vi "ReadFile.vi"(0 "File Path":path, 5 "Error In":errorcluster) -> (14 "file path":path, 15 "Initialize Settings":T1, 16 "Channel(s) Settings":T4 {"Channel(s)"."Verticle Settings"."Vertical Coupling" items=["AC", "DC", "Ground"]; "Channel(s)"."Verticle Settings"."Probe Attenuation" format="%.1f"; "Channel(s)"."Verticle Settings"."Vertical Offset" format="%.2p"; "Channel(s)"."Verticle Settings"."Vertical Range" format="%.2f"; "Channel(s)"."Maximum Input Frequency" format="%.2f"}, 17 "Specific&CommonTriggerProperties":T3={"Common Trigger Settings"={"Trigger Delay"=0.0, "Reference Position"=50.0, "Trigger Modifier"=2, "Auto Triggered"=FALSE}, "Specific Trigger Settings"={"Source"="", "Holdoff"=0.0, "Level"=0.0, "Trigger Slope"=enum."Negative", "Type"=enum."Immediate", "Window Mode"=0, "Low Level"=-0.1, "High Level"=0.1, "Coupling"=1, "Hysteresis"=0.05}} {"Specific Trigger Settings"."Hysteresis" format="%.2f"; "Specific Trigger Settings"."Coupling" items=["AC"=0, "DC"=1, "HF Reject"=3, "LF Reject"=4, "AC Plus HF Reject"=1001]; "Specific Trigger Settings"."High Level" format="%.2f"; "Specific Trigger Settings"."Low Level" format="%.2f"; "Specific Trigger Settings"."Window Mode" items=["Entering", "Leaving"]; "Common Trigger Settings"."Trigger Modifier" items=["None"=1, "Auto Trigger"=2]; "Common Trigger Settings"."Reference Position" format="%.1f"; "Common Trigger Settings"."Trigger Delay" format="%#.4p"}, 18 "Horizontal Settings":T2={"Continuous"=FALSE, "EnableAveraging"=FALSE, "Number Averages"=0, "Measurement Timeout"=0.0, "Min Record Length"=1000, "Min Sample Rate"=10000000.0, "Enforce Realtime"=TRUE, "Sampling Mode "=enum."Real Time", "Interpolation"=enum."No Interpolation", "Type"=enum."Normal", "StartTime"=0.0, "Time Per Record"=0.0, "Number of Points Minimum"=0, "Measurement Name"="Sensor.RoomAlert0", "Measurement RefreshTime (ms)"=1000} {"Min Sample Rate" step=1000000.0 format="%#.2p"}, 19 "error out":errorcluster)   [LabVIEW 2018, in "ScopePlugins.lvlib" / "ScopePluginsBase.lvclass"]
uses:
  ScopePluginsBase.lvclass
  Typedefs/ChannelSetting(s).ctl
  Typedefs/TriggerSettings.ctl
  Typedefs/HorizontalSettings.ctl
  Typedefs/InitializationSettings.ctl
  <vilib>/Utility/config.llb/NI_LVConfig.lvlib
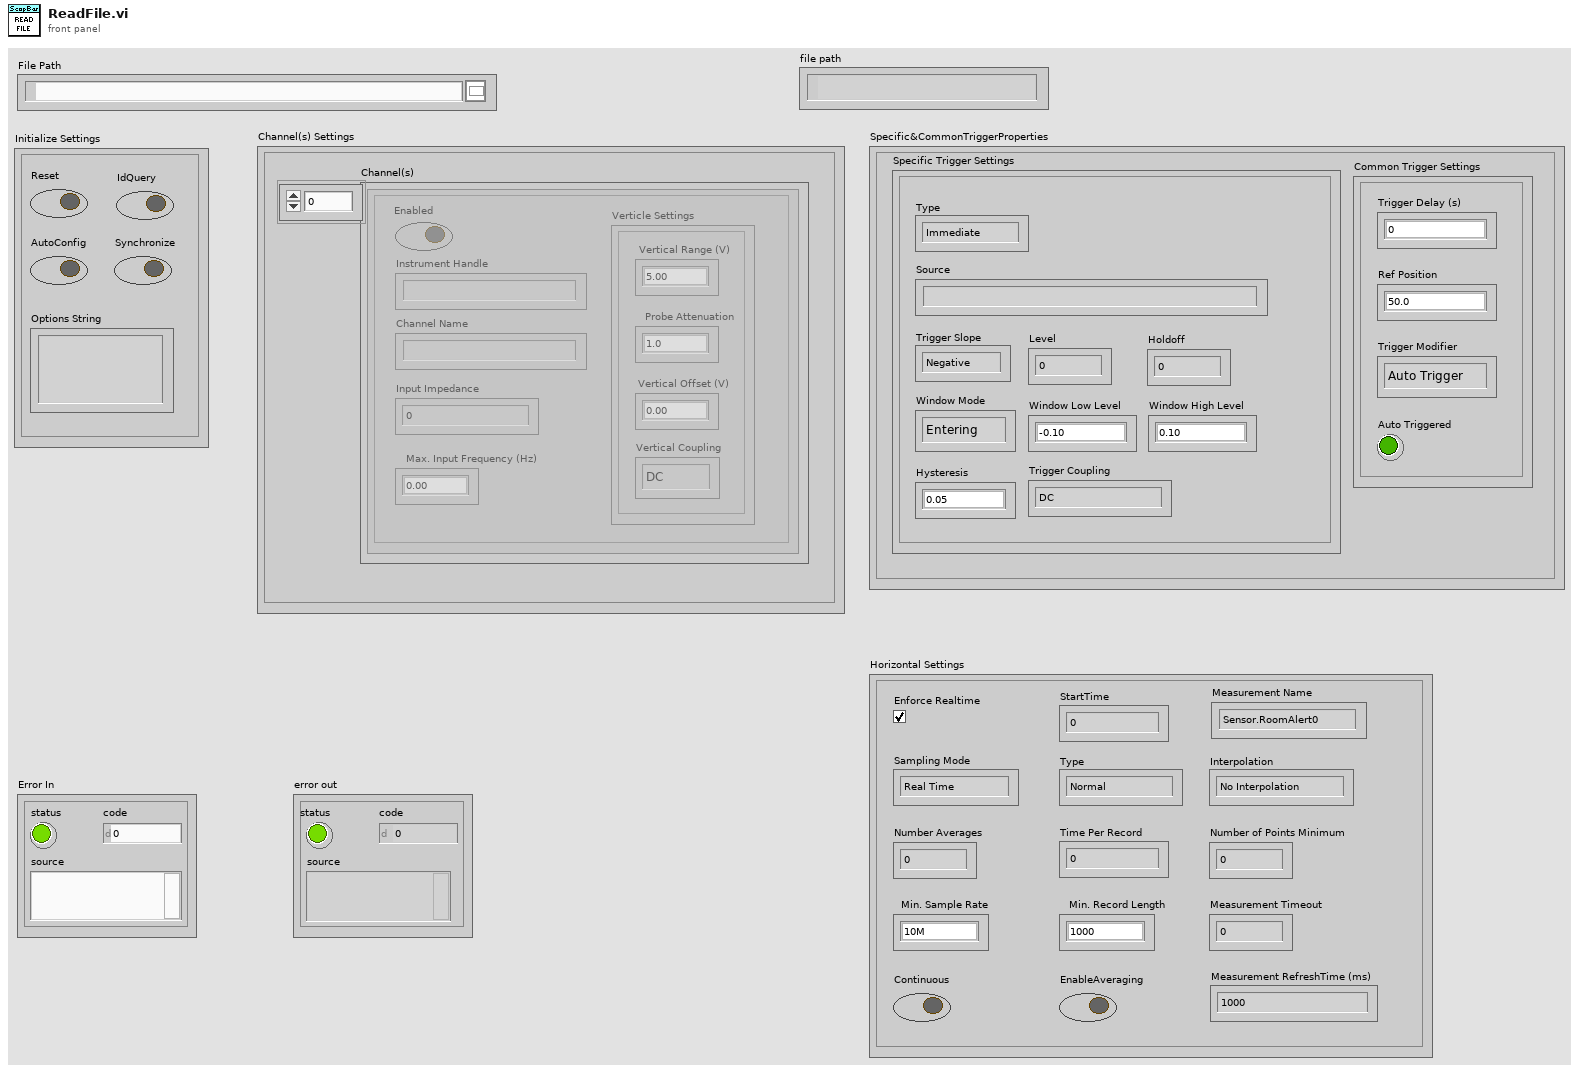
[diagram p1: front panel]
types:
  T1 = typedef "ScopePlugins.lvlib/ScopePluginsBase.lvclass/InitializationSettings.ctl" = cluster{"Reset":bool, "IdQuery":bool, "AutoConfig":bool, "Options String":string, "Synchronize":bool}
  T2 = typedef "ScopePlugins.lvlib/ScopePluginsBase.lvclass/HorizontalSettings.ctl" = cluster{"Continuous":bool, "EnableAveraging":bool, "Number Averages":i32, "Measurement Timeout":dbl, "Min Record Length":i32, "Min Sample Rate":dbl, "Enforce Realtime":bool, "Sampling Mode ":enum16{"Real Time", "Equivalent Time", "Segment", "Real Time Peak Detect", "Real Time High Resolution", "Peak Detect Segment", "High Resolution Segment"}, "Interpolation":enum16{"No Interpolation", "sin(x)/x", "linear", "1 Point sin(x)/x", "2 Point sin(x)/x", "4 Point sin(x)/x", "8 Point sin(x)/x", "16 Point sin(x)/x"}, "Type":enum16{"Normal", "PeakDetect", "HighRes", "Envelope", "Average"}, "StartTime":dbl, "Time Per Record":dbl, "Number of Points Minimum":i32, "Measurement Name":string, "Measurement RefreshTime (ms)":u32}
  T3 = typedef "ScopePlugins.lvlib/ScopePluginsBase.lvclass/TriggerSettings.ctl" = cluster{"Common Trigger Settings":cluster{"Trigger Delay":dbl, "Reference Position":dbl, "Trigger Modifier":i32, "Auto Triggered":bool}, "Specific Trigger Settings":cluster{"Source":string, "Holdoff":dbl, "Level":dbl, "Trigger Slope":enum16{"Negative", "Positive"}, "Type":enum16{"Immediate", "Edge", "Digitial", "Window", "Hysteresis", "Width", "Runt", "Glitch", "TV", "AC Line"}, "Window Mode":i32, "Low Level":dbl, "High Level":dbl, "Coupling":u16, "Hysteresis":dbl}}
  T4 = typedef "ScopePlugins.lvlib/ScopePluginsBase.lvclass/ChannelSetting(s).ctl" = cluster{"Number of Channels":i32, "Channel(s)":cluster{"Enabled":bool, "Instrument Handle":string, "Channel Name":string, "Maximum Input Frequency":dbl, "Verticle Settings":cluster{"Vertical Range":dbl, "Vertical Offset":dbl, "Probe Attenuation":dbl, "Vertical Coupling":i32}, "Connected":bool, "Input Impedance":dbl, "IO Type Instrument Handle":refnum<k15>}[]}
  T5 = typedef "NI_LVConfig.lvlib/Config Data RefNum.ctl" = refnum<k1>
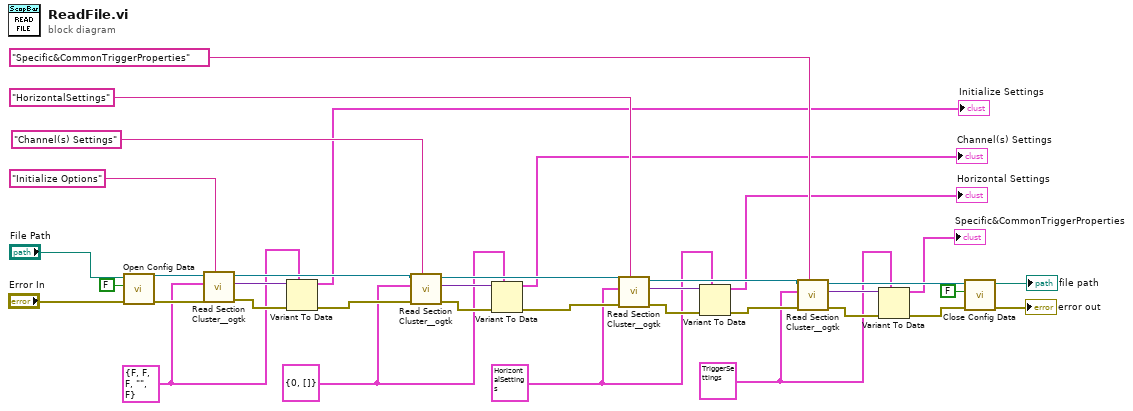
[diagram p0: block diagram]
diagram:
  w1 = T1 {"Reset"=FALSE, "IdQuery"=FALSE, "AutoConfig"=FALSE, "Options String"="", "Synchronize"=FALSE} ("Initialize Settings")
  w6 = T3 {"Common Trigger Settings"={"Trigger Delay"=0.0, "Reference Position"=50.0, "Trigger Modifier"=2, "Auto Triggered"=FALSE}, "Specific Trigger Settings"={"Source"="", "Holdoff"=0.0, "Level"=0.0, "Trigger Slope"=enum."Negative", "Type"=enum."Immediate", "Window Mode"=0, "Low Level"=-0.1, "High Level"=0.1, "Coupling"=1, "Hysteresis"=0.05}} ("Specific&CommonTriggerProperties")
  w7 = T2 {"Continuous"=FALSE, "EnableAveraging"=FALSE, "Number Averages"=0, "Measurement Timeout"=0.0, "Min Record Length"=1000, "Min Sample Rate"=10000000.0, "Enforce Realtime"=TRUE, "Sampling Mode "=enum."Real Time", "Interpolation"=enum."No Interpolation", "Type"=enum."Normal", "StartTime"=0.0, "Time Per Record"=0.0, "Number of Points Minimum"=0, "Measurement Name"="Sensor.RoomAlert0", "Measurement RefreshTime (ms)"=1000} ("Horizontal Settings")
  w8 = T4 {"Number of Channels"=0, "Channel(s)"=[]} ("Channel(s) Settings")
  n1 = call <vilib>:"Open Config Data.vi"("error in (no error)"="Error In", "create file if necessary (T)"=FALSE, "configuration file path"="File Path") -> ("error out"=w30:errorcluster, "refnum"=w29:T5)  [unwired: 6 in, 1 out]
  n2 = call <userlib>:"Read Section Cluster__ogtk.vi"("section (optional)"="Initialize Options", "error in (no error)"=w30, "Section Formatted Cluster Type"=w1, "refnum"=w29) -> ("error out"=w32:errorcluster, "Section Formatted Cluster"=w31:variant, "dup refnum"=w25:T5)  [unwired: 3 in, 2 out]
  n3 = Variant To Data(error in=w32, type=w1, Variant=w31) -> (data=→"Initialize Settings":T1, error out=w24:errorcluster)
  n4 = call <userlib>:"Read Section Cluster__ogtk.vi"("section (optional)"="Channel(s) Settings", "error in (no error)"=w24, "Section Formatted Cluster Type"=w8, "refnum"=w25) -> ("error out"=w26:errorcluster, "Section Formatted Cluster"=w27:variant, "dup refnum"=w20:T5)  [unwired: 3 in, 2 out]
  n5 = Variant To Data(error in=w26, type=w8, Variant=w27) -> (data=→"Channel(s) Settings":T4, error out=w21:errorcluster)
  n6 = call <userlib>:"Read Section Cluster__ogtk.vi"("section (optional)"="HorizontalSettings", "error in (no error)"=w21, "Section Formatted Cluster Type"=w7, "refnum"=w20) -> ("error out"=w23:errorcluster, "Section Formatted Cluster"=w22:variant, "dup refnum"=w14:T5)  [unwired: 3 in, 2 out]
  n7 = Variant To Data(error in=w23, type=w7, Variant=w22) -> (data=→"Horizontal Settings":T2, error out=w15:errorcluster)
  n8 = call <userlib>:"Read Section Cluster__ogtk.vi"("section (optional)"="Specific&CommonTriggerProperties", "error in (no error)"=w15, "Section Formatted Cluster Type"=w6, "refnum"=w14) -> ("error out"=w16:errorcluster, "Section Formatted Cluster"=w17:variant, "dup refnum"=w13:T5)  [unwired: 3 in, 2 out]
  n9 = Variant To Data(error in=w16, type=w6, Variant=w17) -> (data=→"Specific&CommonTriggerProperties":T3, error out=w12:errorcluster)
  n10 = call <vilib>:"Close Config Data.vi"("error in (no error)"=w12, "write file if changed (T)"=FALSE, "refnum"=w13) -> ("error out"=→"error out":errorcluster, "file path"=→"file path":path)  [unwired: 7 in]
